vi "Main.vi"() -> ()   [LabVIEW 2020]
doc: "This template is for the Queued Message Handler design pattern.\n\nThe Event Handling Loop generates messages based on user interface actions.\n\nThe Message Handling Loop processes messages generated by the Event Handling Loop, or by other messages. The messages are string values, so new messages can be added easily to the Message Cases case structure in the Message Handling Loop. Each message cluster can also provide an optional value for Message Data, which is a variant that can be converted to whatever message-specific data is required."
uses:
  controls/keyboard 3x3.ctl
  controls/UI Data.ctl
  controls/General Refnums.ctl
  controls/PlayerSettings.ctl
  controls/PlayerMode.ctl
  controls/Gameplay Data.ctl
  controls/Gameboard Refnums.ctl
  controls/Gameboard Data.ctl
  controls/Player.ctl
  controls/DecisionTree.ctl
  controls/DecisionTreeRecord.ctl
  controls/Message.ctl
  df708d76-7046-4981-afed-609ef43be7ea.vi
  support/Message Queue/Enqueue Message (Single).vi
  <vilib>/Utility/error.llb/Error Cluster From Error Code.vi
  <vilib>/ErrorRing/Error Ring.xnode
  <vilib>/Comparison/Equal/Equal Functor/Equal Functor.lvclass
  support/Message Queue/Message Queue.lvlib
  support/User Event - Stop/User Event - Stop.lvlib
panel:
  in  "Cancel Button":bool
  in  "Settings Button":bool
  in  "Gameboard":T1
  in  "Play Button":bool
  out "Display":string
  in  "Exit":bool
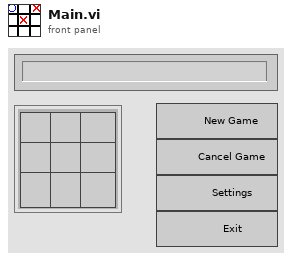
[diagram p1: front panel]
types:
  T1 = typedef "keyboard 3x3.ctl" = cluster{"Button 1":bool, "Button 2":bool, "Button 3":bool, "Button 4":bool, "Button 5":bool, "Button 6":bool, "Button 7":bool, "Button 8":bool, "Button 9":bool}
  T2 = typedef "Gameplay Data.ctl" = cluster{"Gameboard Refs":T3, "Gameboard":T4, "Players":cluster{"Current":cluster{"Player":T5, "Mode":T6}, "Next":cluster{"Player":T5, "Mode":T6}}, "BotDelay (ms)":i32, "DecisionTree":T7}
  T3 = typedef "Gameboard Refnums.ctl" = cluster{"Gameboard":refnum<vi>, "Button Refs":refnum<vi>[]}
  T4 = typedef "Gameboard Data.ctl" = enum16{"None", "Player 1", "Player 2"}[]
  T5 = typedef "Player.ctl" = enum16{"None", "Player 1", "Player 2"}
  T6 = typedef "PlayerMode.ctl" = enum16{"Human", "Bot Random", "Bot Intermidiate", "Bot Perfect Play"}
  T7 = typedef "DecisionTree.ctl" = map{T4, T8}
  T8 = typedef "DecisionTreeRecord.ctl" = cluster{"Status":T5, "GoodMoves":i8[], "MehMoves":i8[], "BadMoves":i8[]}
  T9 = typedef "UI Data.ctl" = cluster{"General Refs":T10, "Settings":T11, "IsGameRunning?":bool}
  T10 = typedef "General Refnums.ctl" = cluster{"Display":refnum<vi>, "Play":refnum<vi>, "Settings":refnum<vi>, "Exit":refnum<vi>, "Cancel":refnum<vi>}
  T11 = typedef "PlayerSettings.ctl" = cluster{"Player 1":T6, "Player 2":T6}
  T12 = enum8{"Enabled", "Disabled", "Disabled and Grayed Out"}
  T13 = typedef "Message Queue.lvlib/All Message Queues.ctl" = cluster{"UI":refnum<queue>, "Players":refnum<queue>}
  T14 = typedef "Message Queue.lvlib/Message.ctl" = enum16{"Update Display", "Initialize", "New Game", "Open Settings", "Cancel Game", "Exit", "Confirm Quit", "Error", "Discard Game", "New Turn", "Human", "Bot Random", "Bot Intermidiate", "Bot Tree", "Apply Move", "Win Conditions", "Game Done"}
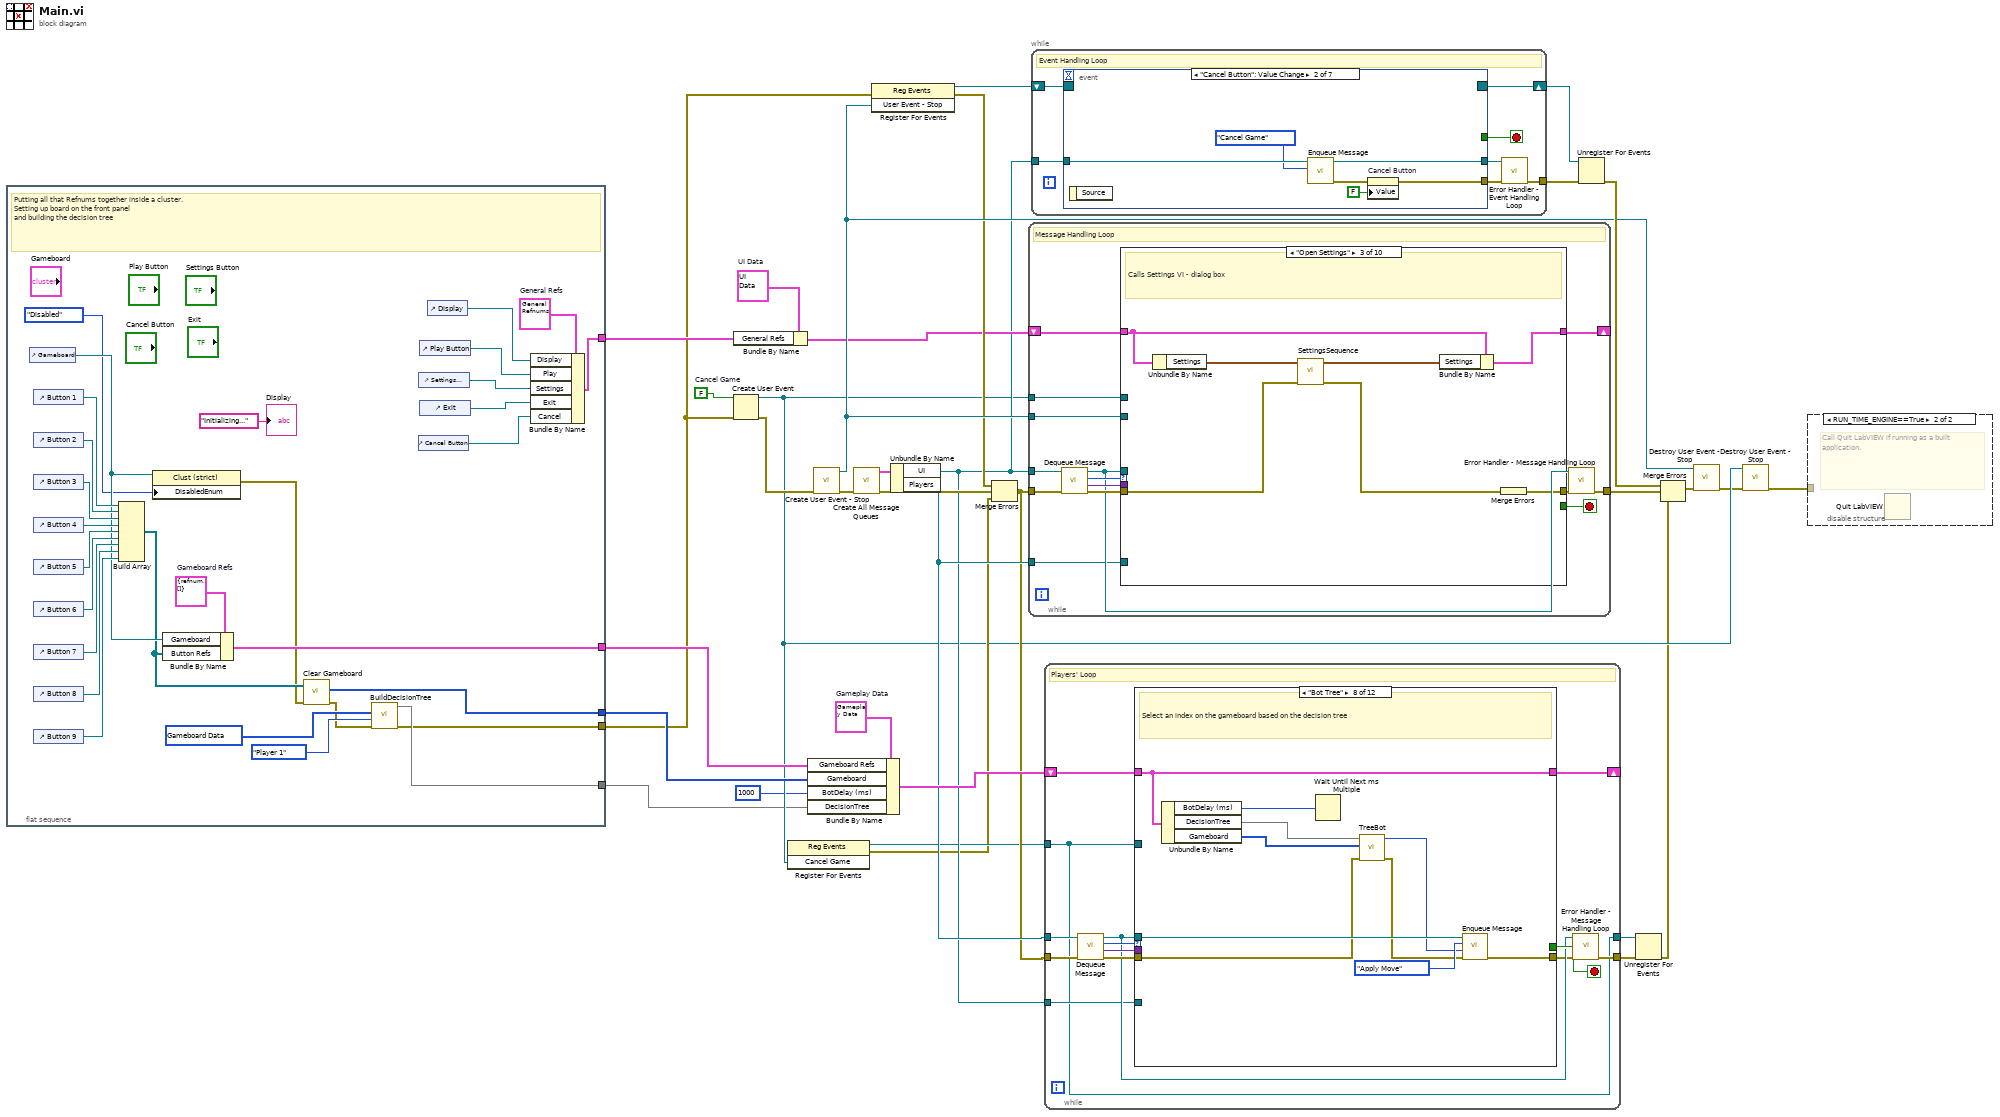
[diagram p0: block diagram]
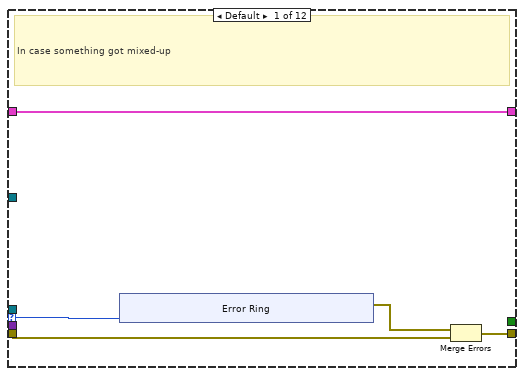
[diagram p2: hidden frame]
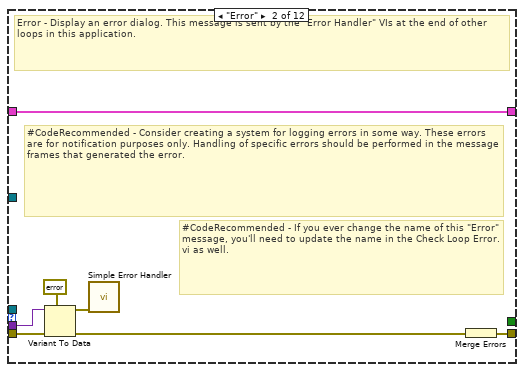
[diagram p3: hidden frame]
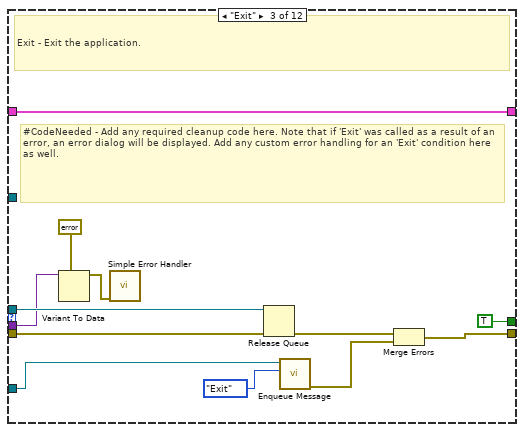
[diagram p4: hidden frame]
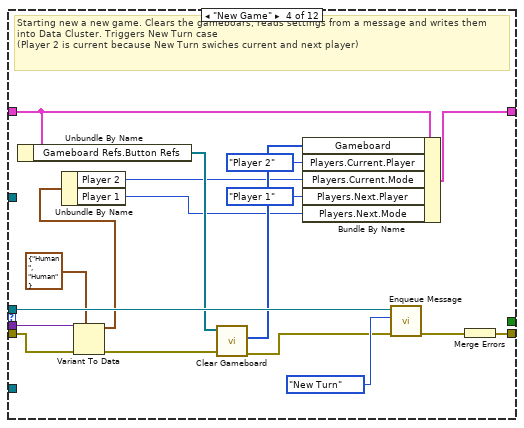
[diagram p5: hidden frame]
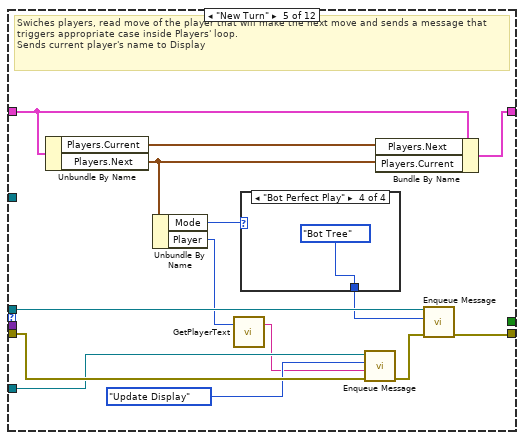
[diagram p6: hidden frame]
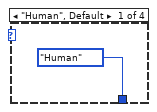
[diagram p7: hidden frame]
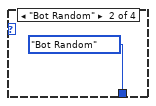
[diagram p8: hidden frame]
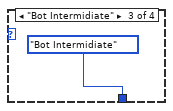
[diagram p9: hidden frame]
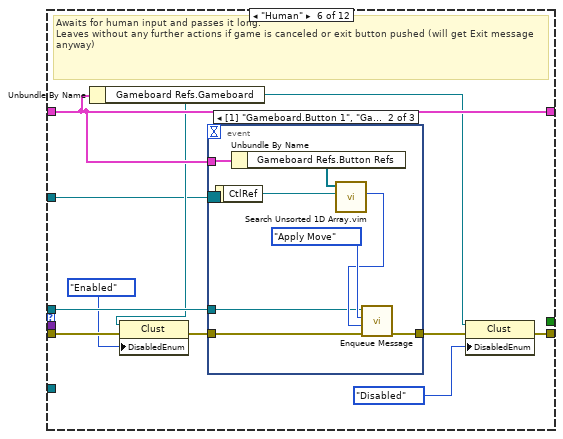
[diagram p10: hidden frame]
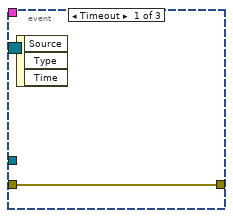
[diagram p11: hidden frame]
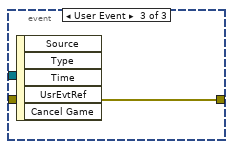
[diagram p12: hidden frame]
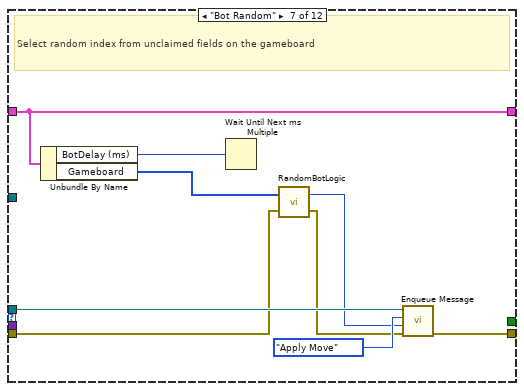
[diagram p13: hidden frame]
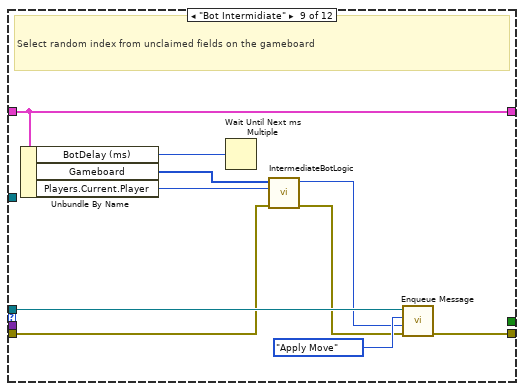
[diagram p14: hidden frame]
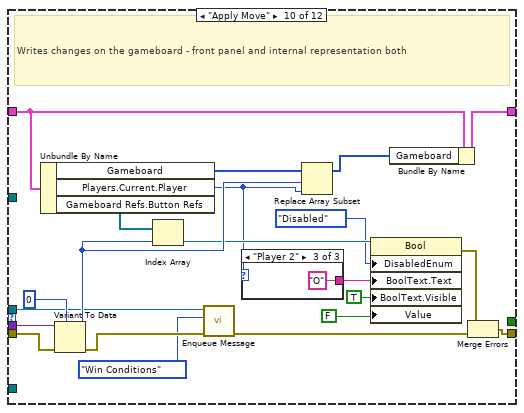
[diagram p15: hidden frame]
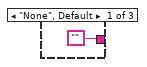
[diagram p16: hidden frame]
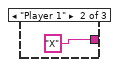
[diagram p17: hidden frame]
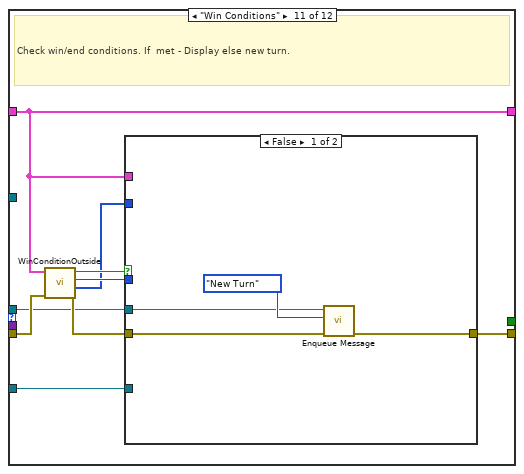
[diagram p18: hidden frame]
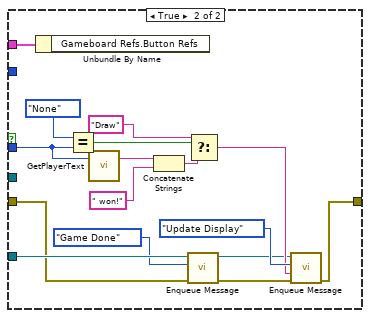
[diagram p19: hidden frame]
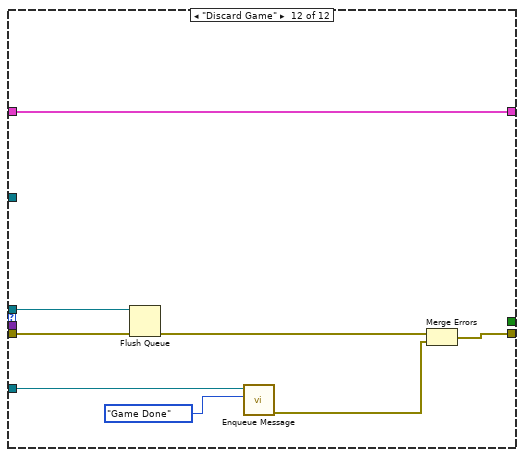
[diagram p20: hidden frame]
diagram:
  w10 = FALSE  # Cancel Game
  w21 = T2 {"Gameboard Refs"={"Gameboard"=refnum, "Button Refs"=[]}, "Gameboard"=[], "Players"={"Current"={"Player"=enum."None", "Mode"=enum."Human"}, "Next"={"Player"=enum."None", "Mode"=enum."Human"}}, "BotDelay (ms)"=0, "DecisionTree"={}}  # Gameplay Data
  w27 = T9 {"General Refs"={"Display"=refnum, "Play"=refnum, "Settings"=refnum, "Exit"=refnum, "Cancel"=refnum}, "Settings"={"Player 1"=enum."Human", "Player 2"=enum."Human"}, "IsGameRunning?"=FALSE}  # UI Data
  n1 = flat-sequence {
    tunnel: [w53] -> w13
    tunnel: [w35] -> w2
    tunnel: [w49] -> w20
    tunnel: [w42] -> w14
    tunnel: [w40] -> w1
    frame #0 {
      w39 = T4 [enum."None", enum."None", enum."None", enum."None", enum."None", enum."None", enum."None", enum."None", enum."None"] items=["None", "Player 1", "Player 2"] ("Gameboard")
      w50 = T10 {"Display"=refnum, "Play"=refnum, "Settings"=refnum, "Exit"=refnum, "Cancel"=refnum}  # General Refs
      w54 = T3 {"Gameboard"=refnum, "Button Refs"=[]}  # Gameboard Refs
      # "Putting all that Refnums together inside a cluster.\nSetting up board on the front panel\nand building the decision tree"
      n2 = control-ref of="Gameboard"() -> (w52:refnum<vi>)
      n3 = control-ref of="Button 1"() -> (w63:refnum<vi>)
      n4 = control-ref of="Button 2"() -> (w62:refnum<vi>)
      n5 = control-ref of="Button 3"() -> (w61:refnum<vi>)
      n6 = control-ref of="Button 4"() -> (w60:refnum<vi>)
      n7 = control-ref of="Button 5"() -> (w59:refnum<vi>)
      n8 = control-ref of="Button 6"() -> (w58:refnum<vi>)
      n9 = control-ref of="Button 7"() -> (w57:refnum<vi>)
      n10 = control-ref of="Button 8"() -> (w56:refnum<vi>)
      n11 = control-ref of="Button 9"() -> (w55:refnum<vi>)
      n12 = Build Array(w63, w62, w61, w60, w59, w58, w57, w56, w55) -> (w44:refnum<vi>[])
      n13 = property class="Clust (strict)"(reference=w52, "DisabledEnum"=T12."Disabled" ("Disabled")) -> (error out=w37:errorcluster)  [unwired: 1 in, 1 out]
      n14 = Bundle By Name(cluster=w54, "Gameboard"=w52, "Button Refs"=w44) -> (w53:T3)
      n15 = call "Clear Gameboard.vi"("error in (no error)"=w37, "Buton Refs IN"=w44) -> ("error out"=w36:errorcluster, "Gameboard"=w42:T4)  [unwired: 8 in]
      n16 = call "BuildDecisionTree.vi"("error in (no error)"=w36, "Current Player"=Player."Player 1", "Gameboard"=w39) -> ("error out"=w35:errorcluster, "DecisionTree Out"=w40:T7)  [unwired: 6 in, 1 out]
      n17 = control-ref of="Cancel Button"() -> (w43:refnum<vi>)
      n18 = control-ref of="Settings Button"() -> (w46:refnum<vi>)
      n19 = control-ref of="Play Button"() -> (w47:refnum<vi>)
      n20 = control-ref of="Exit"() -> (w45:refnum<vi>)
      n21 = control-ref of="Display"() -> (w48:refnum<vi>)
      n22 = Bundle By Name(cluster=w50, "Display"=w48, "Play"=w47, "Settings"=w46, "Exit"=w45, "Cancel"=w43) -> (w49:T10)
      "Display" <- "Initializing..." ("Display")
    }
  }
  n23 = Create User Event(user event datatype=w10, error in=w2) -> (user event=w8:refnum<user-event>, error out=w9:errorcluster)
  n24 = Bundle By Name(cluster=w27, "General Refs"=w20) -> (w22:T9)
  n25 = register-events(w8) -> (reference out=w12:refnum<event-registration>, error out=w11:errorcluster)  [unwired: 2 in]
  n26 = Bundle By Name(cluster=w21, "Gameboard Refs"=w13, "Gameboard"=w14, "BotDelay (ms)"=1000 ("BotDelay"), "DecisionTree"=w1) -> (w19:T2)
  n27 = call "Create User Event - Stop.vi"("error in (no error)"=w9) -> ("error out"=w31:errorcluster, "User Event - Stop"=w24:refnum<user-event>)  [unwired: 9 in]
  n28 = call "Create All Message Queues.vi"("error in (no error)"=w31) -> ("error out"=w34:errorcluster, "Message Queues out"=w33:T13)  [unwired: 9 in]
  n29 = register-events(error in=w2, w24) -> (reference out=w25:refnum<event-registration>, error out=w23:errorcluster)  [unwired: 1 in]
  n30 = Unbundle By Name(w33) -> ("UI"=w16:refnum<queue>, "Players"=w18:refnum<queue>)
  n31 = Merge Errors(w23, w34, w11) -> (w17:errorcluster)
  n32 = while {
    tunnel: w16 -> [w69]
    shift-right: [w76] -> _
    shift-left: w22 -> [w77]
    tunnel: w24 -> [w74]
    tunnel: w17 -> [w73]
    tunnel: [w67] -> w32
    tunnel: w18 -> [w65]
    tunnel: w8 -> [w64]
    stop <- w75 stop-if-true
    # "Message Handling Loop"
    n33 = call "Dequeue Message.vi"("error in (no error)"=w73, "Message Queue"=w69) -> ("error out"=w72:errorcluster, "Message Data"=w70:variant, "Message"=w71:T14, "dup Message Queue"=w68:refnum<queue>)  [unwired: 6 in]
    n34 = case "Message Cases" shown="\"Open Settings\"" w71 {
      selector: w71 -> [_ _ _ _ _ _ _ _ _ w180]
      tunnel: w68 -> [w82 w91 _ w120 _ _ _ w158 w179 _]
      tunnel: w72 -> [w85 w87 w109 w115 w139 w147 w155 w162 w172 w181]
      tunnel: [w86 w92 w114 w121 w139 w148 w149 w160 w175 w183] -> w66
      tunnel: w77 -> [w84 w89 w113 w117 w138 w143 w154 w161 w178 w184]
      tunnel: [w80 w90 w110 w117 w137 w143 w154 w161 w178 w184] -> w76
      tunnel: [_ _ _ _ _ _ _ _ TRUE _] -> w75
      tunnel: w70 -> [_ _ _ _ _ w146 w153 _ w169 _]
      tunnel: w74 -> [_ _ _ _ _ _ _ _ w174 _]
      tunnel: w65 -> [_ w93 _ w118 _ _ _ _ w167 _]
      tunnel: w64 -> [_ _ _ w116 _ _ _ _ w165 _]
      frame "Initialize" {
        # "Initialize - All initialization work should take place in this message, since other loops can potentially enqueue messages that execute immediately after this one."
        n35 = Bundle By Name(cluster=w84, "Settings"=T11 {"Player 1"=enum."Human", "Player 2"=enum."Bot Intermidiate"}, "IsGameRunning?"=FALSE) -> (w80:T9)
        n36 = call-poly "Enqueue Message.vi"("error in (no error)"=w85, "Message Data"="Ready. Press New Game to play", "Message"=Message."Update Display", "Message Queue"=w82) -> ("error out"=w86:errorcluster)  [unwired: 6 in, 1 out]
      }
      frame "New Game" {
        # "Something - Replace this message with functionality for your own application."
        n37 = Unbundle By Name(w89) -> ("IsGameRunning?"=w88:bool)
        n38 = case shown="False" w88 {
          tunnel: w93 -> [w105 _]
          tunnel: [w104 w106] -> w92
          tunnel: w89 -> [w94 w107]
          tunnel: w87 -> [w101 w106]
          tunnel: w91 -> [w99 _]
          tunnel: [w96 w107] -> w90
          frame False {
            n39 = Unbundle By Name(w94) -> ("Settings"=w102:T11)
            n40 = Bundle By Name(cluster=w94, "IsGameRunning?"=TRUE) -> (w96:T9)
            n41 = call-poly "Enqueue Message.vi"("error in (no error)"=w101, "Message Data"="", "Message"=Message."Update Display", "Message Queue"=w99) -> ("error out"=w100:errorcluster)  [unwired: 6 in, 1 out]
            n42 = call-poly "Enqueue Message.vi"("error in (no error)"=w100, "Message Data"=w102, "Message"=Message."New Game", "Message Queue"=w105) -> ("error out"=w104:errorcluster)  [unwired: 6 in, 1 out]
          }
          frame True {
          }
        }
      }
      frame "Open Settings" {
        # "Calls Settings VI - dialog box"
        n43 = Unbundle By Name(w113) -> ("Settings"=w112:T11)
        n44 = call "SettingsSequence.vi"("error in (no error)"=w109, "Settings"=w112) -> ("error out"=w108:errorcluster, "Settings out"=w111:T11)  [unwired: 8 in]
        n45 = Bundle By Name(cluster=w113, "Settings"=w111) -> (w110:T9)
        n46 = Merge Errors(w108) -> (w114:errorcluster)
      }
      frame "Cancel Game" {
        # "If game is running send messages to discard it"
        n47 = Unbundle By Name(w117) -> ("IsGameRunning?"=w119:bool)
        n48 = case shown="True" w119 {
          tunnel: w115 -> [w122 w135]
          tunnel: [w122 w124] -> w121
          tunnel: w120 -> [_ w134]
          tunnel: w118 -> [_ w129]
          tunnel: w116 -> [_ w125]
          frame False {
          }
          frame True {
            n49 = Generate User Event(user event=w125, event data cluster=TRUE ("event data")) -> (error out=w123:errorcluster)  [unwired: 2 in, 1 out]
            n50 = call-poly "Enqueue Message.vi"("error in (no error)"=w135, "Message Data"="Game Canceled. Press New Game to play", "Message"=Message."Update Display", "Message Queue"=w134) -> ("error out"=w130:errorcluster)  [unwired: 6 in, 1 out]
            n51 = call-poly "Enqueue Message.vi"("Priority Message? (F)"=TRUE, "error in (no error)"=w130, "Message"=Message."Discard Game", "Message Queue"=w129) -> ("error out"=w131:errorcluster)  [unwired: 6 in, 1 out]
            n52 = Merge Errors(w123, w131) -> (w124:errorcluster)
          }
        }
      }
      frame "Game Done" {
        n53 = Bundle By Name(cluster=w138, "IsGameRunning?"=FALSE) -> (w137:T9)
      }
      frame "Update Display" {
        # "Update Display - Convert the message data to a string to display in the Data Display indicator."
        n54 = Unbundle By Name(w143) -> ("General Refs.Display"=w142:refnum<vi>)
        n55 = Variant To Data(error in=w147, type="", Variant=w146) -> (data=w141:string, error out=w144:errorcluster)
        n56 = property class="Str"(reference=w142, "Value"=w141) -> (error out=w140:errorcluster)  [unwired: 1 in, 1 out]
        n57 = Merge Errors(w140, w144) -> (w148:errorcluster)
      }
      frame "Error" {
        # "#CodeRecommended - If you ever change the name of this \"Error\" message, you'll need to update the name in the Check Loop Error.vi as well."
        # "#CodeRecommended - Consider creating a system for logging errors in some way. These errors are for notification purposes only. Handling of specific errors should be performed in the message frames that generated the error."
        # "Error - Display an error dialog. This message is sent by the \"Error Handler\" VIs at the end of other loops in this application."
        n58 = Variant To Data(error in=w155, type=errorcluster {"status"=FALSE, "code"=0, "source"=""} ("error constant"), Variant=w153) -> (data=w151:errorcluster, error out=w150:errorcluster)
        n59 = call <vilib>:"Simple Error Handler.vi"("error in (no error)"=w151) -> ()  [unwired: 4 in, 5 out]
        n60 = Merge Errors(w150) -> (w149:errorcluster)
      }
      frame "Confirm Quit" {
        # "#CodeNeeded - If you want to provide an \"Are you sure\" dialog (or some other notification) before the application exits, place that code here. This message is typically sent from a Panel Close? event."
        # "Confirm Quit - Message that can confirm whether or not the user wants to exit the application."
        n61 = call-poly "Enqueue Message.vi"("Priority Message? (F)"=TRUE, "error in (no error)"=w162, "Message"=Message."Exit", "Message Queue"=w158) -> ("error out"=w159:errorcluster)  [unwired: 6 in, 1 out]
        n62 = Merge Errors(w159) -> (w160:errorcluster)
      }
      frame "Exit" {
        # "#CodeNeeded - Add any required cleanup code here. Note that if 'Exit' was called as a result of an error, an error dialog will be displayed. Add any custom error handling for an 'Exit' condition here as well."
        # "Exit - Exit the application."
        n63 = Variant To Data(type=errorcluster {"status"=FALSE, "code"=0, "source"=""} ("error constant"), Variant=w169) -> (data=w170:errorcluster)  [unwired: 1 in, 1 out]
        n64 = call <vilib>:"Simple Error Handler.vi"("error in (no error)"=w170) -> ()  [unwired: 4 in, 5 out]
        n65 = Generate User Event(user event=w165, event data cluster=TRUE ("event data")) -> (error out=w163:errorcluster)  [unwired: 2 in, 1 out]
        n66 = call "Fire User Event - Stop.vi"("error in (no error)"=w163, "User Event - Stop"=w174) -> ("error out"=w173:errorcluster)  [unwired: 9 in]
        n67 = Release Queue(queue=w179, error in (no error)=w172) -> (error out=w176:errorcluster)  [unwired: 1 in, 2 out]
        n68 = call-poly "Enqueue Message.vi"("Message"=Message."Exit", "Message Queue"=w167) -> ("error out"=w168:errorcluster)  [unwired: 8 in, 1 out]
        n69 = Merge Errors(w173, w176, w168) -> (w175:errorcluster)
      }
      frame Default {
        # "In case something got mixed-up"
        n70 = xnode "Error Ring"("parameter 0"=w180) -> ("error out"=w182:errorcluster)
        n71 = Merge Errors(w182, w181) -> (w183:errorcluster)
      }
    }
    n72 = call "Error Handler - Message Handling Loop.vi"("error in (no error)"=w66, "Message Queue"=w68) -> ("dup error in"=w67:errorcluster)  [unwired: 8 in, 1 out]
  }
  n73 = while {
    tunnel: w16 -> [w198]
    shift-right: [w196] -> w28
    shift-left: w25 -> [w197]
    tunnel: [w192] -> w26
    stop <- w194 stop-if-true
    # "Event Handling Loop"
    n74 = event shown="[1] \"Cancel Button\": Value Change" {
      selector: w197 -> [_ _ _ _ _ _ _]
      dyn-events: [_ _ _ _ _ _ _] -> w196
      timeout: _ -> [_ _ _ _ _ _ _]
      tunnel: [_ _ _ _ _ _ TRUE ("Discard?")] -> w194
      tunnel: w198 -> [w204 w210 w214 w219 w221 w228 w231]
      tunnel: [w200 w205 w212 w218 _ w223 _] -> w195
      tunnel: [w203 w209 w213 w217 w221 w227 w231] -> w193
      event "Play Button": Value Change {
        n75 = event-data() -> ()  [unwired: 1 in, 1 out]
        n76 = call-poly "Enqueue Message.vi"("Message"=Message."New Game", "Message Queue"=w204) -> ("error out"=w199:errorcluster, "dup Message Queue"=w203:refnum<queue>)  [unwired: 8 in]
        n77 = property on="Play Button" class="Bool (strict)"(error in=w199, "Value"=FALSE ("Play Button")) -> (error out=w200:errorcluster)  [unwired: 1 in, 1 out]
      }
      event "Cancel Button": Value Change {
        n78 = event-data() -> ()  [unwired: 1 in, 1 out]
        n79 = call-poly "Enqueue Message.vi"("Message"=Message."Cancel Game", "Message Queue"=w210) -> ("error out"=w206:errorcluster, "dup Message Queue"=w209:refnum<queue>)  [unwired: 8 in]
        n80 = property on="Cancel Button" class="Bool (strict)"(error in=w206, "Value"=FALSE ("Play Button")) -> (error out=w205:errorcluster)  [unwired: 1 in, 1 out]
      }
      event "Settings Button": Value Change {
        n81 = event-data() -> ()  [unwired: 1 in, 1 out]
        n82 = call-poly "Enqueue Message.vi"("Message"=Message."Open Settings", "Message Queue"=w214) -> ("error out"=w212:errorcluster, "dup Message Queue"=w213:refnum<queue>)  [unwired: 8 in]
      }
      event Panel Close? {
        # "Send the 'Confirm Quit' message if the user closes the panel of the VI. Discard the event so the 'Confirm Quit' message has a chance to run."
        n83 = event-data() -> ()  [unwired: 1 in, 1 out]
        n84 = call-poly "Enqueue Message.vi"("Priority Message? (F)"=TRUE, "Message"=Message."Confirm Quit", "Message Queue"=w219) -> ("error out"=w218:errorcluster, "dup Message Queue"=w217:refnum<queue>)  [unwired: 7 in]
        n85 = event-data("Discard?"=TRUE) -> ()  [unwired: 1 in, 1 out]
      }
      event Application Instance Close {
        # "#CodeRecommended - When a project closes, all VIs within that project are aborted and leave memory. However, any code placed in this event frame is guaranteed to run to completion, so add any cleanup code that absolutely must happen here."
        n86 = event-data() -> ()  [unwired: 1 in, 1 out]
      }
      event "Exit": Value Change {
        n87 = event-data() -> ()  [unwired: 1 in, 1 out]
        n88 = call-poly "Enqueue Message.vi"("Priority Message? (F)"=TRUE, "Message"=Message."Exit", "Message Queue"=w228) -> ("error out"=w224:errorcluster, "dup Message Queue"=w227:refnum<queue>)  [unwired: 7 in]
        n89 = property on="Exit" class="Bool (strict)"(error in=w224, "Value"=FALSE ("Exit")) -> (error out=w223:errorcluster)  [unwired: 1 in, 1 out]
      }
      event User Event {
        # "The Message Handling Loop processed an \"Exit\" message, which fired this event to stop the Event Handling Loop."
        n90 = event-data() -> ()  [unwired: 1 in, 1 out]
        n91 = property on="Display" class="Str"("Text.Text"="") -> ()  [unwired: 2 in, 2 out]
      }
    }
    n92 = call "Error Handler - Event Handling Loop.vi"("error in (no error)"=w195, "Message Queue"=w193) -> ("dup error in"=w192:errorcluster)  [unwired: 8 in, 1 out]
  }
  n93 = while {
    tunnel: w18 -> [w237]
    shift-right: [w243] -> _
    shift-left: w19 -> [w244]
    tunnel: w17 -> [w241]
    tunnel: [w235] -> w15
    tunnel: w16 -> [w233]
    tunnel: w12 -> [w232]
    tunnel: [w232] -> w4
    stop <- w242 stop-if-true
    # "Players' Loop"
    n94 = call "Dequeue Message.vi"("error in (no error)"=w241, "Message Queue"=w237) -> ("error out"=w240:errorcluster, "Message Data"=w238:variant, "Message"=w239:T14, "dup Message Queue"=w236:refnum<queue>)  [unwired: 6 in]
    n95 = case "Message Cases" shown="\"Bot Tree\"" w239 {
      selector: w239 -> [w245 _ _ _ _ _ _ _ _ _ _ _]
      tunnel: w236 -> [_ _ w275 w291 w299 w321 w339 w349 w359 w363 w386 w420]
      tunnel: w240 -> [w246 w263 w270 w284 w302 w319 w333 w345 w352 w381 w392 w419]
      tunnel: [w248 w257 w271 w293 w300 w316 w340 w350 w360 w367 w391 w416] -> w234
      tunnel: w244 -> [w249 w262 w274 w287 w307 w320 w336 w347 w356 w378 w385 w421]
      tunnel: [w249 w262 w274 w286 w306 w320 w336 w347 w356 w374 w385 w421] -> w243
      tunnel: [_ _ TRUE _ _ _ _ _ _ _ _ _] -> w242
      tunnel: w238 -> [_ w261 w267 w282 _ _ _ _ _ w380 _ _]
      tunnel: w233 -> [_ _ w265 _ w298 _ _ _ _ _ w390 w417]
      tunnel: w232 -> [_ _ _ _ _ w312 _ _ _ _ _ _]
      frame Default {
        # "In case something got mixed-up"
        n96 = xnode "Error Ring"("parameter 0"=w245) -> ("error out"=w247:errorcluster)
        n97 = Merge Errors(w247, w246) -> (w248:errorcluster)
      }
      frame "Error" {
        # "#CodeRecommended - If you ever change the name of this \"Error\" message, you'll need to update the name in the Check Loop Error.vi as well."
        # "#CodeRecommended - Consider creating a system for logging errors in some way. These errors are for notification purposes only. Handling of specific errors should be performed in the message frames that generated the error."
        # "Error - Display an error dialog. This message is sent by the \"Error Handler\" VIs at the end of other loops in this application."
        n98 = Variant To Data(error in=w263, type=errorcluster {"status"=FALSE, "code"=0, "source"=""} ("error constant"), Variant=w261) -> (data=w259:errorcluster, error out=w258:errorcluster)
        n99 = call <vilib>:"Simple Error Handler.vi"("error in (no error)"=w259) -> ()  [unwired: 4 in, 5 out]
        n100 = Merge Errors(w258) -> (w257:errorcluster)
      }
      frame "Exit" {
        # "#CodeNeeded - Add any required cleanup code here. Note that if 'Exit' was called as a result of an error, an error dialog will be displayed. Add any custom error handling for an 'Exit' condition here as well."
        # "Exit - Exit the application."
        n101 = Variant To Data(type=errorcluster {"status"=FALSE, "code"=0, "source"=""} ("error constant"), Variant=w267) -> (data=w268:errorcluster)  [unwired: 1 in, 1 out]
        n102 = call <vilib>:"Simple Error Handler.vi"("error in (no error)"=w268) -> ()  [unwired: 4 in, 5 out]
        n103 = Release Queue(queue=w275, error in (no error)=w270) -> (error out=w272:errorcluster)  [unwired: 1 in, 2 out]
        n104 = call-poly "Enqueue Message.vi"("Message"=Message."Exit", "Message Queue"=w265) -> ("error out"=w266:errorcluster)  [unwired: 8 in, 1 out]
        n105 = Merge Errors(w272, w266) -> (w271:errorcluster)
      }
      frame "New Game" {
        # "Starting new a new game. Clears the gameboars, reads settings from a message and writes them into Data Cluster. Triggers New Turn case\n(Player 2 is current because New Turn swiches current and next player)"
        n106 = Unbundle By Name(w287) -> ("Gameboard Refs.Button Refs"=w289:refnum<vi>[])
        n107 = Variant To Data(error in=w284, type=T11 {"Player 1"=enum."Human", "Player 2"=enum."Human"} ("Settings"), Variant=w282) -> (data=w280:T11, error out=w283:errorcluster)
        n108 = Unbundle By Name(w280) -> ("Player 2"=w278:T6, "Player 1"=w279:T6)
        n109 = call "Clear Gameboard.vi"("error in (no error)"=w283, "Buton Refs IN"=w289) -> ("error out"=w288:errorcluster, "Gameboard"=w285:T4)  [unwired: 8 in]
        n110 = Bundle By Name(cluster=w287, "Gameboard"=w285, "Players.Current.Player"=Player."Player 2", "Players.Current.Mode"=w278, "Players.Next.Player"=Player."Player 1", "Players.Next.Mode"=w279) -> (w286:T2)
        n111 = call-poly "Enqueue Message.vi"("error in (no error)"=w288, "Message"=Message."New Turn", "Message Queue"=w291) -> ("error out"=w292:errorcluster)  [unwired: 7 in, 1 out]
        n112 = Merge Errors(w292) -> (w293:errorcluster)
      }
      frame "New Turn" {
        # "Swiches players, read move of the player that will make the next move and sends a message that triggers appropriate case inside Players' loop.\nSends current player's name to Display"
        n113 = Unbundle By Name(w307) -> ("Players.Current"=w305:cluster{"Player":T5, "Mode":T6}, "Players.Next"=w304:cluster{"Player":T5, "Mode":T6})
        n114 = Unbundle By Name(w304) -> ("Mode"=w303:T6, "Player"=w295:T5)
        n115 = call "GetPlayerText.vi"("Player"=w295) -> ("Text"=w294:string)  [unwired: 2 in]
        n116 = case shown="\"Bot Perfect Play\"" w303 {
          tunnel: [Message."Human" ("Message") Message."Bot Random" ("Message") Message."Bot Intermidiate" ("Message") Message."Bot Tree" ("Message")] -> w297
          frame "Human", Default {
          }
          frame "Bot Random" {
          }
          frame "Bot Intermidiate" {
          }
          frame "Bot Perfect Play" {
          }
        }
        n117 = call-poly "Enqueue Message.vi"("error in (no error)"=w302, "Message Data"=w294, "Message"=Message."Update Display", "Message Queue"=w298) -> ("error out"=w301:errorcluster)  [unwired: 6 in, 1 out]
        n118 = Bundle By Name(cluster=w307, "Players.Next"=w305, "Players.Current"=w304) -> (w306:T2)
        n119 = call-poly "Enqueue Message.vi"("error in (no error)"=w301, "Message"=w297, "Message Queue"=w299) -> ("error out"=w300:errorcluster)  [unwired: 7 in, 1 out]
      }
      frame "Human" {
        # "Awaits for human input and passes it long.\nLeaves without any further actions if game is canceled or exit button pushed (will get Exit message anyway)"
        n120 = Unbundle By Name(w320) -> ("Gameboard Refs.Gameboard"=w315:refnum<vi>)
        n121 = property class="Clust"(reference=w315, error in=w319, "DisabledEnum"=T12."Enabled" ("Disabled")) -> (error out=w318:errorcluster)  [unwired: 1 out]
        n122 = event shown="[1] \"Gameboard.Button 1\", \"Gameboard.Button 2\", \"Gameboard.Button 3\", \"Gameboard.Button 4\", \"Gameboard.Button 5\", \"Gameboard.Button 6\", \"Gameboard.Button 7\", \"Gameboard.Button 8\", \"Gameboard.Button 9\": Value Change" {
          selector: w312 -> [_ _ _]
          dyn-events: _ -> [_ _ _]
          timeout: _ -> [_ _ _]
          tunnel: w320 -> [_ w330 _]
          tunnel: [w322 w325 w331] -> w317
          tunnel: w318 -> [w322 w323 w331]
          tunnel: w321 -> [_ w326 _]
          event Timeout {
            n123 = event-data() -> ()  [unwired: 1 in, 3 out]
          }
          event Value Change {
            n124 = event-data() -> ("CtlRef"=w324:refnum<vi>)  [unwired: 1 in]
            n125 = Unbundle By Name(w330) -> ("Gameboard Refs.Button Refs"=w329:refnum<vi>[])
            n126 = call "Search Unsorted 1D Array.vim"("element"=w324, "unsorted 1D array"=w329) -> ("index of element"=w327:i32)  [unwired: 9 in]
            n127 = call-poly "Enqueue Message.vi"("error in (no error)"=w323, "Message Data"=w327, "Message"=Message."Apply Move", "Message Queue"=w326) -> ("error out"=w325:errorcluster)  [unwired: 6 in, 1 out]
          }
          event User Event {
            n128 = event-data() -> ()  [unwired: 1 in, 5 out]
          }
        }
        n129 = property class="Clust"(reference=w315, error in=w317, "DisabledEnum"=T12."Disabled" ("Disabled")) -> (error out=w316:errorcluster)  [unwired: 1 out]
      }
      frame "Bot Random" {
        # "Select random index from unclaimed fields on the gameboard"
        n130 = Unbundle By Name(w336) -> ("BotDelay (ms)"=w334:i32, "Gameboard"=w335:T4)
        n131 = Wait Until Next ms Multiple(millisecond multiple=w334) -> ()  [unwired: 1 out]
        n132 = call "RandomBotLogic.vi"("error in (no error)"=w333, "Gameboard"=w335) -> ("error out"=w332:errorcluster, "Selected Index"=w337:i8)
        n133 = call-poly "Enqueue Message.vi"("error in (no error)"=w332, "Message Data"=w337, "Message"=Message."Apply Move", "Message Queue"=w339) -> ("error out"=w340:errorcluster)  [unwired: 6 in, 1 out]
      }
      frame "Bot Tree" {
        # "Select an index on the gameboard based on the decision tree"
        n134 = Unbundle By Name(w347) -> ("BotDelay (ms)"=w346:i32, "DecisionTree"=w342:T7, "Gameboard"=w341:T4)
        n135 = Wait Until Next ms Multiple(millisecond multiple=w346) -> ()  [unwired: 1 out]
        n136 = call "TreeBot.vi"("error in (no error)"=w345, "Gameboard"=w341, "Map"=w342) -> ("error out"=w344:errorcluster, "Move"=w343:i8)  [unwired: 7 in]
        n137 = call-poly "Enqueue Message.vi"("error in (no error)"=w344, "Message Data"=w343, "Message"=Message."Apply Move", "Message Queue"=w349) -> ("error out"=w350:errorcluster)  [unwired: 6 in, 1 out]
      }
      frame "Bot Intermidiate" {
        # "Select random index from unclaimed fields on the gameboard"
        n138 = Unbundle By Name(w356) -> ("BotDelay (ms)"=w354:i32, "Gameboard"=w355:T4, "Players.Current.Player"=w353:T5)
        n139 = Wait Until Next ms Multiple(millisecond multiple=w354) -> ()  [unwired: 1 out]
        n140 = call "IntermediateBotLogic.vi"("error in (no error)"=w352, "Current Player"=w353, "Gameboard"=w355) -> ("error out"=w351:errorcluster, "Selected Index"=w357:i8)  [unwired: 6 in, 1 out]
        n141 = call-poly "Enqueue Message.vi"("error in (no error)"=w351, "Message Data"=w357, "Message"=Message."Apply Move", "Message Queue"=w359) -> ("error out"=w360:errorcluster)  [unwired: 6 in, 1 out]
      }
      frame "Apply Move" {
        # "Writes changes on the gameboard - front panel and internal representation both"
        n142 = Unbundle By Name(w378) -> ("Gameboard"=w377:T4, "Players.Current.Player"=w370:T5, "Gameboard Refs.Button Refs"=w375:refnum<vi>[])
        n143 = Variant To Data(error in=w381, type=0, Variant=w380) -> (data=w376:i32, error out=w365:errorcluster)
        n144 = Index Array(array=w375, index=w376) -> (element=w372:refnum<vi>)
        n145 = call-poly "Enqueue Message.vi"("error in (no error)"=w365, "Message"=Message."Win Conditions", "Message Queue"=w363) -> ("error out"=w364:errorcluster)  [unwired: 7 in, 1 out]
        n146 = case shown="\"Player 2\"" w370 {
          tunnel: ["" "X" "O"] -> w369
          frame "None", Default {
          }
          frame "Player 1" {
          }
          frame "Player 2" {
          }
        }
        n147 = Replace Array Subset(array=w377, new element=w370, index=w376) -> (w373:T4)
        n148 = property class="Bool"(reference=w372, "DisabledEnum"=T12."Disabled" ("Disabled"), "BoolText.Text"=w369, "BoolText.Visible"=TRUE ("Boolean Text.Visible"), "Value"=FALSE) -> (error out=w366:errorcluster)  [unwired: 1 in, 1 out]
        n149 = Bundle By Name(cluster=w378, "Gameboard"=w373) -> (w374:T2)
        n150 = Merge Errors(w366, w364) -> (w367:errorcluster)
      }
      frame "Win Conditions" {
        # "Check win/end conditions. If  met - Display else new turn."
        n151 = call "WinConditionOutside.vi"("error in (no error)"=w392, "Gameplay Data"=w385) -> ("error out"=w389:errorcluster, "LineIndices"=w387:i8[], "Winner"=w388:T5, "End?"=w393:bool)  [unwired: 6 in]
        n152 = case shown="False" w393 {
          tunnel: [w394 w413] -> w391
          tunnel: w390 -> [_ w402]
          tunnel: w389 -> [w395 w399]
          tunnel: w388 -> [_ w408]
          tunnel: w387 -> [_ _]
          tunnel: w386 -> [w396 _]
          tunnel: w385 -> [_ w406]
          frame False {
            n153 = call-poly "Enqueue Message.vi"("error in (no error)"=w395, "Message"=Message."New Turn", "Message Queue"=w396) -> ("error out"=w394:errorcluster)  [unwired: 7 in, 1 out]
          }
          frame True {
            n154 = Unbundle By Name(w406) -> ()  [unwired: 1 out]
            n155 = Equal?(x=Player."None" ("Player"), y=w408) -> (x = y?=w410:bool)
            n156 = call "GetPlayerText.vi"("Player"=w408) -> ("Text"=w404:string)  [unwired: 2 in]
            n157 = Concatenate Strings(w404, " won!") -> (w405:string)
            n158 = call-poly "Enqueue Message.vi"("error in (no error)"=w399, "Message"=Message."Game Done", "Message Queue"=w402) -> ("error out"=w400:errorcluster, "dup Message Queue"=w401:refnum<queue>)  [unwired: 7 in]
            n159 = Select(t="Draw", s=w410, f=w405) -> (s? t:f=w407:string)
            n160 = call-poly "Enqueue Message.vi"("error in (no error)"=w400, "Message Data"=w407, "Message"=Message."Update Display", "Message Queue"=w401) -> ("error out"=w413:errorcluster)  [unwired: 6 in, 1 out]
          }
        }
      }
      frame "Discard Game" {
        n161 = Flush Queue(queue=w420, error in (no error)=w419) -> (error out=w418:errorcluster)  [unwired: 2 out]
        n162 = call-poly "Enqueue Message.vi"("Message"=Message."Game Done", "Message Queue"=w417) -> ("error out"=w415:errorcluster)  [unwired: 8 in, 1 out]
        n163 = Merge Errors(w418, w415) -> (w416:errorcluster)
      }
    }
    n164 = call "Error Handler - Message Handling Loop.vi"("error in (no error)"=w234, "Message Queue"=w236) -> ("dup error in"=w235:errorcluster)  [unwired: 8 in, 1 out]
  }
  n165 = Unregister For Events(event registration refnum=w28, error in=w26) -> (error out=w29:errorcluster)
  n166 = Unregister For Events(event registration refnum=w4, error in=w15) -> (error out=w5:errorcluster)
  n167 = Merge Errors(w29, w32, w5) -> (w30:errorcluster)
  n168 = call "Destroy User Event - Stop.vi"("error in (no error)"=w30, "User Event - Stop"=w24) -> ("error out"=w7:errorcluster)  [unwired: 9 in]
  n169 = call "Destroy User Event - Stop.vi"("error in (no error)"=w7, "User Event - Stop"=w8) -> ("error out"=w6:errorcluster)  [unwired: 9 in]
  n170 = disable-structure shown="RUN_TIME_ENGINE==True" {
    disable-tunnel: w6 -> [_ _]
    frame condition #0 (active) {
    }
    frame condition #1 {
      # "Call Quit LabVIEW if running as a built application."
      n171 = Quit LabVIEW() -> ()  [unwired: 1 in]
    }
  }
